vi "picoStatus.vi"(1 "PICO STATUS":i32, 2 "error in":errorcluster, 3 "source":string) -> (0 "error out":errorcluster)   [LabVIEW 2011]
doc: "This VI checks the status value returned by calls to the driver. If the driver returns an error, the status member of the error cluster is set to 'true' and the error code and source are set."
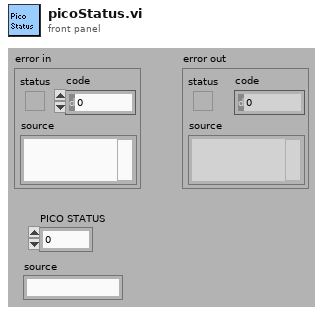
[diagram p1: front panel]
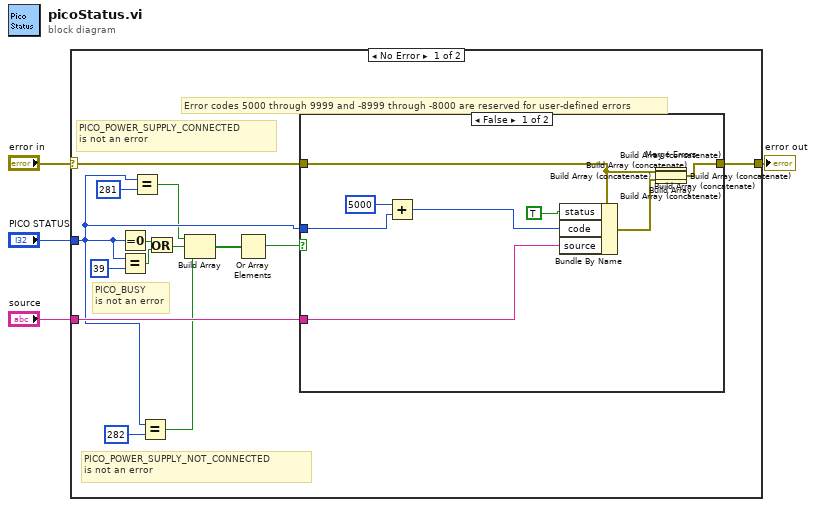
[diagram p0: block diagram]
diagram:
  n1 = case shown="No Error" "error in" {
    selector: "error in" -> [w17 w35]
    tunnel: [w18 w35] -> w4
    tunnel: "PICO STATUS" -> [w10 _]
    tunnel: "source" -> [w16 _]
    frame No Error {
      # "PICO_POWER_SUPPLY_CONNECTED \nis not an error"
      # "PICO_POWER_SUPPLY_NOT_CONNECTED \nis not an error"
      # "PICO_BUSY \nis not an error"
      # "Error codes 5000 through 9999 and -8999 through -8000 are reserved for user-defined errors"
      n2 = Equal To 0?(x=w10) -> (x = 0?=w15:bool)
      n3 = Equal?(x=w10, y=39) -> (x = y?=w14:bool)
      n4 = Equal?(x=w10, y=281) -> (x = y?=w9:bool)
      n5 = Equal?(x=w10, y=282) -> (x = y?=w7:bool)
      n6 = Or(x=w15, y=w14) -> (x .or. y?=w8:bool)
      n7 = Build Array(w9, w8, w7) -> (w6:bool[])
      n8 = Or Array Elements(Boolean array=w6) -> (logical OR=w5:bool)
      n9 = case shown="False" w5 {
        tunnel: w17 -> [w32 w34]
        tunnel: [w33 w34] -> w18
        tunnel: w10 -> [w31 _]
        tunnel: w16 -> [w26 _]
        frame False {
          n10 = Add(x=5000, y=w31) -> (x+y=w27:i32)
          n11 = Bundle By Name(cluster=w32, "status"=TRUE, "code"=w27, "source"=w26) -> (w30:errorcluster)
          n12 = Build Array(w32, w30) -> (w25:errorcluster[])
          n13 = Build Array (concatenate)(w25) -> (w24:errorcluster[])
          n14 = Build Array (concatenate)(w24) -> (w23:errorcluster[])
          n15 = Build Array (concatenate)(w23) -> (w22:errorcluster[])
          n16 = Build Array (concatenate)(w22) -> (w21:errorcluster[])
          n17 = Build Array (concatenate)(w21) -> (w20:errorcluster[])
          n18 = Build Array (concatenate)(w20) -> (w19:errorcluster[])
          n19 = Merge Errors(w19) -> (w33:errorcluster)
        }
        frame True {
        }
      }
    }
    frame Error {
    }
  }
  "error out" <- w4
